vi "Dialog Option.vi"(9 "Dialog?":bool, 11 "Save File in":refnum<class "Save File.lvclass">) -> (3 "Save File out":refnum<class "Save File.lvclass">)   [LabVIEW 2018, in "Save File Actor.lvlib" / "Save File.lvclass"]
doc: "Let's you select whether or not to pop up a dialog box to select the path and file name to save as."
uses:
  Save File.lvclass
  Save File.lvclass/Save File.ctl
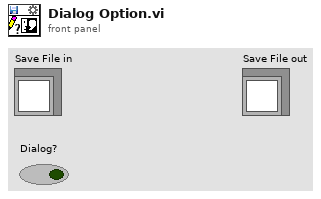
[diagram p1: front panel]
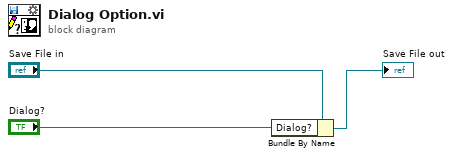
[diagram p0: block diagram]
diagram:
  n1 = Bundle By Name(cluster="Save File in", "Dialog?"="Dialog?") -> (→"Save File out":refnum<class "Save File.lvclass">)
